vi "rpm calibration.vi"(11 "RPM Calibration":T1) -> (2 "STAMP intercept":dbl, 3 "STAMP slope":dbl=1.0)   [LabVIEW 2012]
uses:
  <vilib>/Analysis/NI_AALPro.lvlib
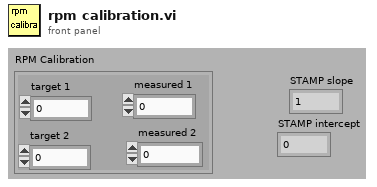
[diagram p1: front panel]
types:
  T1 = cluster{"target 1":dbl, "target 2":dbl, "measured 1":dbl, "measured 2":dbl}
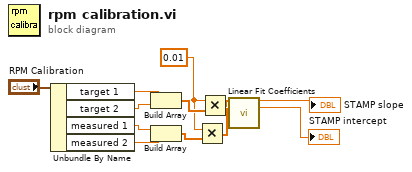
[diagram p0: block diagram]
diagram:
  w1 = 0.01 ("slope")
  n1 = Unbundle By Name("RPM Calibration") -> ("target 1"=w12:dbl, "target 2"=w11:dbl, "measured 1"=w10:dbl, "measured 2"=w9:dbl)
  n2 = Build Array(w12, w11) -> (w6:dbl[])
  n3 = Build Array(w10, w9) -> (w5:dbl[])
  n4 = Multiply(x=w1, y=w5) -> (x*y=w2:dbl[])
  n5 = Multiply(x=w1, y=w6) -> (x*y=w3:dbl[])
  n6 = call <vilib>:"Linear Fit Coefficients.vi"("Y"=w3, "X"=w2) -> ("slope"=→"STAMP slope":dbl, "intercept"=→"STAMP intercept":dbl)  [unwired: 11 in, 1 out]
